vi "PH_IEEE1394Camera.ask serial number.vi"(2 "IMAQ1394 Session In":T1, 4 "Cam Error in":errorcluster) -> (16 "IMAQ1394 Session Out":T1, 17 "Serial Number":dbl, 18 "Cam Error out":errorcluster)   [LabVIEW 2014, in "PH_IEEE1394Camera.lvlib"]
doc: "This VI asks the connected cam for the serial number."
uses:
  PH_IEEE1394Camera.lvlib
  <vilib>/userdefined/High Color/IMAQdx.ctl
  <resource>/objmgr/imaqdx.rc
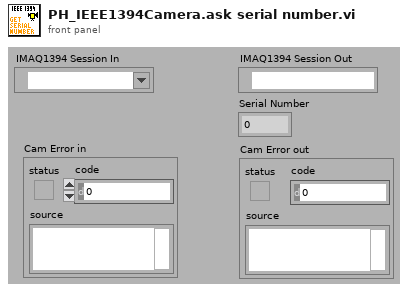
[diagram p1: front panel]
types:
  T1 = typedef "IMAQdx.ctl" = refnum<k21>
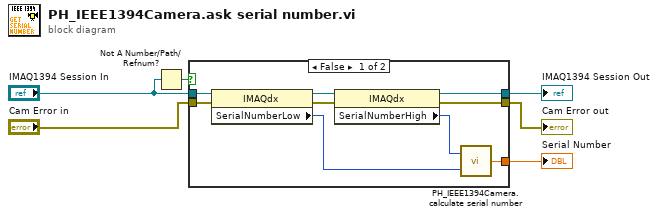
[diagram p0: block diagram]
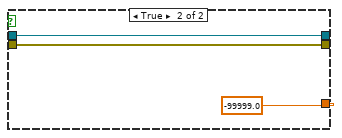
[diagram p2: hidden frame]
diagram:
  n1 = Not A Number/Path/Refnum?(number/path/refnum="IMAQ1394 Session In") -> (NaN/Path/Refnum?=w4:bool)
  n2 = case shown="False" w4 {
    tunnel: "IMAQ1394 Session In" -> [w13 w18]
    tunnel: [w12 w18] -> w1
    tunnel: "Cam Error in" -> [w11 w17]
    tunnel: [w10 -99999.0] -> w5
    tunnel: [w9 w17] -> w6
    frame False {
      n3 = property class="IMAQdx"(reference=w13, error in=w11) -> (reference out=w15:T1, error out=w14:errorcluster, "SerialNumberLow"=w8:u32)
      n4 = property class="IMAQdx"(reference=w15, error in=w14) -> (reference out=w12:T1, error out=w9:errorcluster, "SerialNumberHigh"=w7:u32)
      n5 = call "PH_IEEE1394Camera.calculate serial number.vi"("SerialNumberLow"=w8, "SerialNumberHigh"=w7) -> ("Serial Number"=w10:dbl)
    }
    frame True {
    }
  }
  "Cam Error out" <- w6
  "Serial Number" <- w5
  "IMAQ1394 Session Out" <- w1
